vi "Init.vi"(8 "error in (no error)":errorcluster, 9 "PositionIndCtrls":T2, 10 "MotionStatusCtrls":T1) -> (0 "error out":errorcluster, 3 "UI MotionStatus out":refnum<class "UI MotionStatus.lvclass">)   [LabVIEW 2019, in "UI MotionStatus.lvclass"]
doc: "store control refs for updating the UI\ninit controls"
uses:
  UI MotionStatus.lvclass
  PositonIndicatorsCtrlRefs.ctl
  MotionStatusLEDCtrlRefs.ctl
  UI MotionStatus.lvclass/UI MotionStatus.ctl
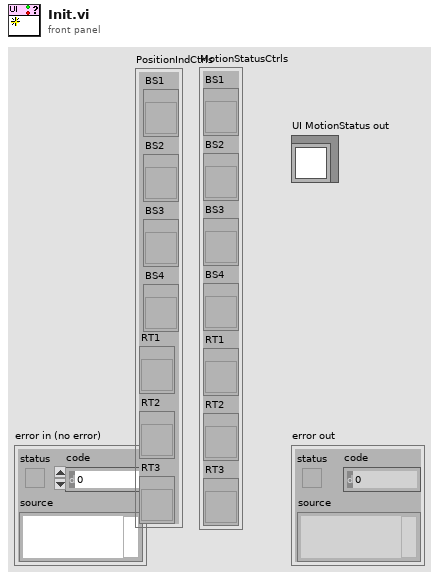
[diagram p1: front panel]
types:
  T1 = typedef "MotionStatusLEDCtrlRefs.ctl" = cluster{"BS1":refnum<vi>, "BS2":refnum<vi>, "BS3":refnum<vi>, "BS4":refnum<vi>, "RT1":refnum<vi>, "RT2":refnum<vi>, "RT3":refnum<vi>}
  T2 = typedef "PositonIndicatorsCtrlRefs.ctl" = cluster{"BS1":refnum<vi>, "BS2":refnum<vi>, "BS3":refnum<vi>, "BS4":refnum<vi>, "RT3":refnum<vi>, "RT2":refnum<vi>, "RT1":refnum<vi>}
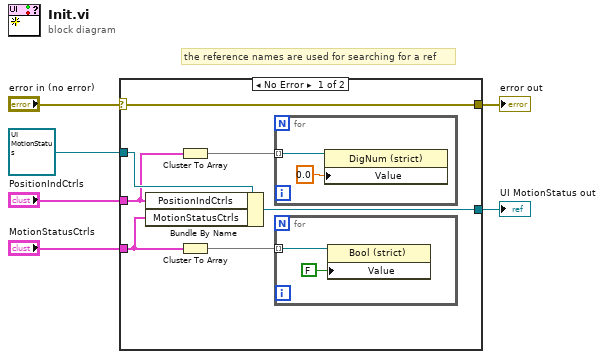
[diagram p0: block diagram]
diagram:
  # "the reference names are used for searching for a ref"
  n1 = case shown="No Error" "error in (no error)" {
    selector: "error in (no error)" -> [w12 w19]
    tunnel: [w12 w19] -> w5
    tunnel: [w11 w18] -> w3
    tunnel: refnum<class "UI MotionStatus.lvclass"> refnum ("UI MotionStatus in") -> [w13 w18]
    tunnel: "PositionIndCtrls" -> [w10 _]
    tunnel: "MotionStatusCtrls" -> [w9 _]
    frame No Error {
      n2 = Bundle By Name(cluster=w13, "PositionIndCtrls"=w10, "MotionStatusCtrls"=w9) -> (w11:refnum<class "UI MotionStatus.lvclass">)
      n3 = Cluster To Array(cluster=w10) -> (array=w8:refnum<vi>[])
      n4 = Cluster To Array(cluster=w9) -> (array=w7:refnum<vi>[])
      n5 = for {
        tunnel: w8 -> [w17] mode=indexing
        n6 = property class="DigNum (strict)"(reference=w17, "Value"=sgl 0.0) -> ()  [unwired: 1 in, 2 out]
      }
      n7 = for {
        tunnel: w7 -> [w15] mode=indexing
        n8 = property class="Bool (strict)"(reference=w15, "Value"=FALSE) -> ()  [unwired: 1 in, 2 out]
      }
    }
    frame Error {
    }
  }
  "error out" <- w5
  "UI MotionStatus out" <- w3
